vi "path_init.vi"(7 "Main vi's path":path) -> (2 "Ini path":path, 3 "Stripped path":path)   [LabVIEW 2018]
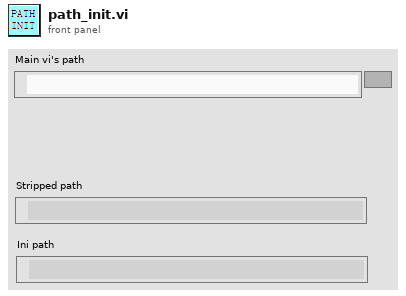
[diagram p1: front panel]
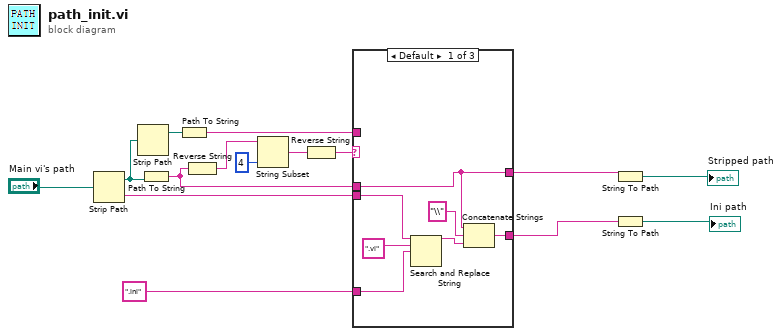
[diagram p0: block diagram]
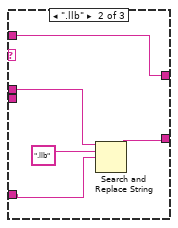
[diagram p2: hidden frame]
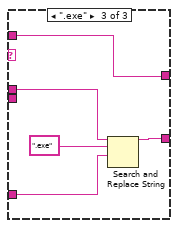
[diagram p3: hidden frame]
diagram:
  n1 = Strip Path(path="Main vi's path") -> (stripped path=w15:path, name=w10:string)
  n2 = Strip Path(path=w15) -> (stripped path=w14:path)  [unwired: 1 out]
  n3 = Path To String(path=w15) -> (string=w7:string)
  n4 = Path To String(path=w14) -> (string=w8:string)
  n5 = Reverse String(1:w7) -> (0:w6:string)
  n6 = String Subset(string=w6, length (rest)=4 ("length (rest)")) -> (substring=w4:string)  [unwired: 1 in]
  n7 = Reverse String(1:w4) -> (0:w3:string)
  n8 = case shown="Default" w3 {
    tunnel: w10 -> [w20 _ _]
    tunnel: ".ini" ("substring (\"\")") -> [w21 w27 w32]
    tunnel: [w16 w24 w29] -> w2
    tunnel: [w17 w25 w30] -> w1
    tunnel: w8 -> [_ w25 w30]
    tunnel: w7 -> [w17 w23 w28]
    frame Default {
      n9 = Search and Replace String(input string=w20, search string=".vi" ("substring (\"\")"), replace string=w21) -> (result string=w18:string)  [unwired: 5 in, 3 out]
      n10 = Concatenate Strings(w17, "\\", w18) -> (w16:string)
    }
    frame ".llb" {
      n11 = Search and Replace String(input string=w23, search string=".llb", replace string=w27) -> (result string=w24:string)  [unwired: 5 in, 3 out]
    }
    frame ".exe" {
      n12 = Search and Replace String(input string=w28, search string=".exe", replace string=w32) -> (result string=w29:string)  [unwired: 5 in, 3 out]
    }
  }
  n13 = String To Path(string=w1) -> (path=→"Stripped path":path)
  n14 = String To Path(string=w2) -> (path=→"Ini path":path)
